vi "Test Code.vi"() -> ()   [LabVIEW 2011]
uses:
  CardInfo/SPR_01.vi
panel:
  out "found 2":bool
  out "found":bool
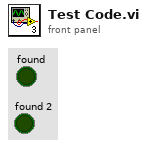
[diagram p1: front panel]
types:
  T1 = enum16{"Initial", "Insert", "Delete", "Search", "Release"}
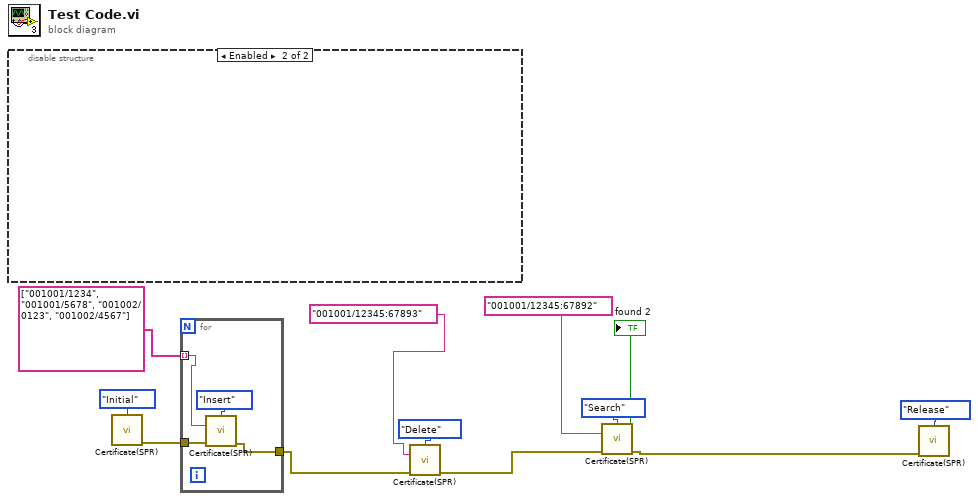
[diagram p0: block diagram]
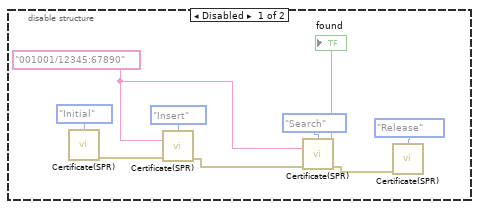
[diagram p2: hidden frame]
diagram:
  n1 = disable-structure shown="Enabled" {
    frame Disabled {
      w15 = "001001/12345:67890" ("key")
      n2 = call-poly "Certificate(SPR).vi"("select"=T1."Initial") -> ("error out"=w17:errorcluster)  [unwired: 12 in, 2 out]
      n3 = call-poly "Certificate(SPR).vi"("select"=T1."Insert", "key"=w15, "error in"=w17) -> ("error out"=w16:errorcluster)  [unwired: 10 in, 2 out]
      n4 = call-poly "Certificate(SPR).vi"("select"=T1."Search", "key"=w15, "error in"=w16) -> ("found"=→"found":bool, "error out"=w13:errorcluster)  [unwired: 10 in, 1 out]
      n5 = call-poly "Certificate(SPR).vi"("select"=T1."Release", "error in"=w13) -> ()  [unwired: 11 in, 3 out]
    }
    frame Enabled {
    }
  }
  n6 = call-poly "Certificate(SPR).vi"("select"=T1."Initial") -> ("error out"=w10:errorcluster)  [unwired: 12 in, 2 out]
  n7 = for {
    tunnel: [w25] -> w4
    tunnel: w10 -> [w24]
    tunnel: string[] ["001001/1234", "001001/5678", "001002/0123", "001002/4567"] -> [w22] mode=indexing
    n8 = call-poly "Certificate(SPR).vi"("select"=T1."Insert", "key"=w22, "error in"=w24) -> ("error out"=w25:errorcluster)  [unwired: 10 in, 2 out]
  }
  n9 = call-poly "Certificate(SPR).vi"("select"=T1."Delete", "key"="001001/12345:67893", "error in"=w4) -> ("error out"=w3:errorcluster)  [unwired: 10 in, 2 out]
  n10 = call-poly "Certificate(SPR).vi"("select"=T1."Search", "key"="001001/12345:67892", "error in"=w3) -> ("found"=→"found 2":bool, "error out"=w12:errorcluster)  [unwired: 10 in, 1 out]
  n11 = call-poly "Certificate(SPR).vi"("select"=T1."Release", "error in"=w12) -> ()  [unwired: 11 in, 3 out]
